vi "Close_SMU's.vi"(8 "Error In":errorcluster, 11 "Instrument_Visas":T1) -> (0 "Error Out":errorcluster)   [LabVIEW 2013]
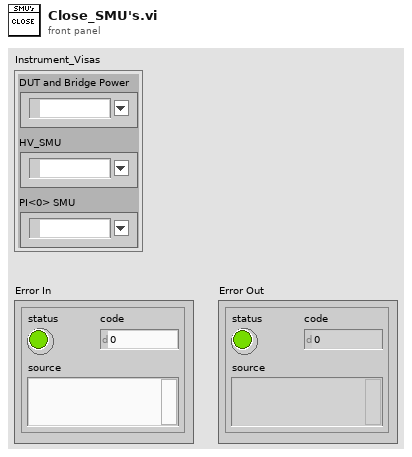
[diagram p1: front panel]
types:
  T1 = cluster{"DUT and Bridge Power":refnum<k15>, "HV_SMU":refnum<k15>, "PI<0> SMU":refnum<k15>}
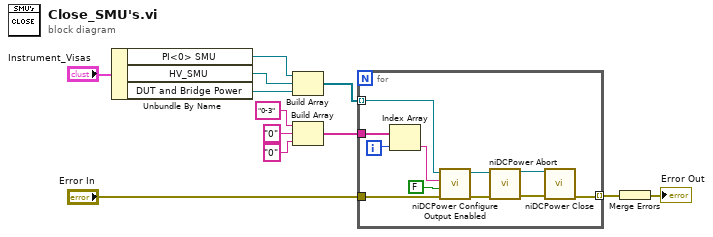
[diagram p0: block diagram]
diagram:
  n1 = Unbundle By Name("Instrument_Visas") -> ("PI<0> SMU"=w11:refnum<k15>, "HV_SMU"=w10:refnum<k15>, "DUT and Bridge Power"=w9:refnum<k15>)
  n2 = Build Array(w11, w10, w9) -> (w8:refnum<k15>[])
  n3 = Build Array("0-3" ("channels"), "0" ("channels"), "0" ("channels")) -> (w4:string[])
  n4 = for {
    tunnel: w8 -> [w19] mode=indexing
    tunnel: w4 -> [w18]
    tunnel: "Error In" -> [w14]
    tunnel: [w13] -> w2 mode=indexing
    i -> [w17]
    n5 = Index Array(array=w18, index=w17) -> (element=w16:string)
    n6 = call <instrlib>:"niDCPower Configure Output Enabled.vi"("error in (no error)"=w14, "output enabled"=FALSE, "channel name"=w16, "instrument handle"=w19) -> ("error out"=w23:errorcluster, "instrument handle out"=w22:refnum<k15>)  [unwired: 6 in]
    n7 = call <instrlib>:"niDCPower Abort.vi"("error in (no error)"=w23, "instrument handle"=w22) -> ("error out"=w21:errorcluster, "instrument handle out"=w20:refnum<k15>)  [unwired: 8 in]
    n8 = call <instrlib>:"niDCPower Close.vi"("error in (no error)"=w21, "instrument handle"=w20) -> ("error out"=w13:errorcluster)  [unwired: 9 in]
  }
  n9 = Merge Errors(w2) -> (→"Error Out":errorcluster)
